vi "简易角度与弧度转换器.vi"() -> ()   [LabVIEW 2012, in "几何工具.lvlib"]
uses:
  Deg to Rad(dbl).vi
  Rad to Deg(dbl)L.vi
panel:
  in  "停止":bool
  in  "Mode":enum16{"Deg to Rad", "Rad to Deg"}(ring)
  out "Output":dbl
  in  "Input":dbl
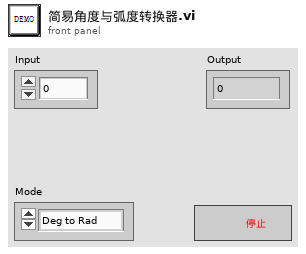
[diagram p1: front panel]
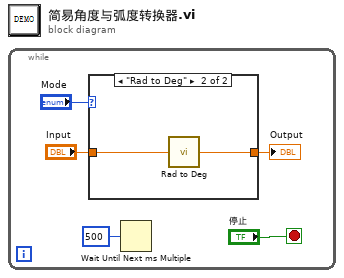
[diagram p0: block diagram]
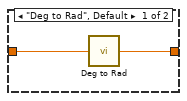
[diagram p2: hidden frame]
diagram:
  n1 = while {
    stop <- "停止" stop-if-true
    n2 = case shown="\"Rad to Deg\"" "Mode" {
      tunnel: "Input" -> [w7 w9]
      tunnel: [w6 w8] -> w3
      frame "Deg to Rad", Default {
        n3 = call-poly "Deg to Rad.vi"("degree"=w7) -> ("radian"=w6:dbl)
      }
      frame "Rad to Deg" {
        n4 = call-poly "Rad to Deg.vi"("radian"=w9) -> ("degree"=w8:dbl)
      }
    }
    "Output" <- w3
    n5 = Wait Until Next ms Multiple(millisecond multiple=u32 500 ("毫秒倍数")) -> ()  [unwired: 1 out]
  }
